vi "Create Default Attributes.vi"(5 "Unique ID":string, 7 "Process Executive Ref":refnum<data-value>, 11 "Start Under Body Wash in":refnum<class "Start Under Body Wash.lvclass">) -> (3 "Start Under Body Wash out":refnum<class "Start Under Body Wash.lvclass">)   [LabVIEW 2019, in "Start Under Body Wash.lvclass"]
uses:
  <vilib>/gpm_packages/@cs/Car-wash/Source/Process Steps/Start Under Body Wash/Start Under Body Wash.lvclass
  <vilib>/gpm_packages/@cs/test-executive/Source/Test Executive/ITestExecutive/ITest Executive.lvclass
  26735e7a-1674-4b69-9c11-14fd20e014ce.vi
  <vilib>/Utility/error.llb/Error Cluster From Error Code.vi
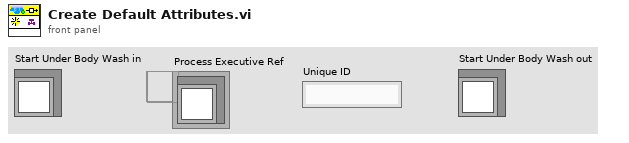
[diagram p1: front panel]
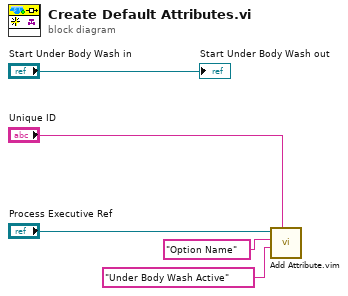
[diagram p0: block diagram]
diagram:
  n1 = call "Add Attribute.vim"("ID"="Unique ID", "Attribute"="Under Body Wash Active" ("Item Name"), "Attribute Name"="Option Name" ("Item Name"), "Test Executive Ref"="Process Executive Ref") -> ()  [unwired: 4 in, 4 out]
  "Start Under Body Wash out" <- "Start Under Body Wash in"
